vi "MicroZed Test Bench.vi"() -> ()   [LabVIEW 2014]
uses:
  Controls/NamedError.ctl
  Controls/PC Data.ctl
  Controls/MicroZed Config Op Mode.ctl
  Controls/MicroZed Config.ctl
panel:
  out "Version String":string
  in  "PC Config":T1={"AC Voltage SP"=0.0, "AC Current SP"=0.0, "Frequency SP"=60.0, "DC Voltage SP"=0.0, "Op Mode SP"=enum."Shutdown (Reset)", "Clear Faults SP"=0} {"Clear Faults SP" format="%01x"; "DC Voltage SP" min=300 max=550 format="%2.1f"; "Frequency SP" min=45 max=65 format="%2.1f"; "AC Current SP" min=-500 max=500 format="%2.1f"; "AC Voltage SP" min=0 max=132 format="%2.1f"}
  out "PC Data":T3 {"Alarms 2" format="%016b"; "Faults 2" format="%016b"; "Alarms 1" format="%016b"; "Faults 1" format="%016b"; "Contactor FB" format="%.0b"; "DC Voltage SP" format="%2.1f"; "Clear Faults SP" format="%.0b"; "Neutral Current" format="%2.1f"; "AC Current - L2" format="%2.1f"; "AC Voltage - L2" format="%2.1f"; "Temperature" format="%2.1f"; "DC Voltage" format="%2.1f"; "AC Current SP" format="%2.1f"; "AC Voltage SP" format="%2.1f"; "Frequency SP" format="%2.1f"; "AC Frequency" format="%2.1f"; "AC Current - L1" format="%2.1f"; "AC Voltage- L1" format="%2.1f"}
  out "Counter":i32
  in  "port (502)":u16=1502
  in  "address":string="192.168.1.231"
  in  "Clear Error":bool
  out "Slave Error":T4
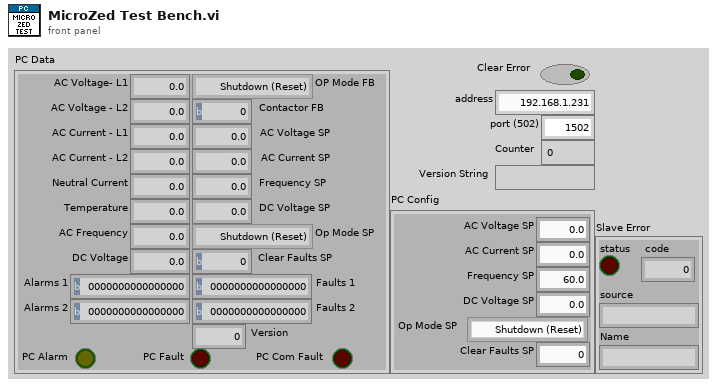
[diagram p1: front panel]
types:
  T1 = typedef "MicroZed Config.ctl" = cluster{"AC Voltage SP":sgl, "AC Current SP":sgl, "Frequency SP":sgl, "DC Voltage SP":sgl, "Op Mode SP":T2, "Clear Faults SP":i16}
  T2 = typedef "MicroZed Config Op Mode.ctl" = enum16{"Shutdown (Reset)", "Startup", "Idle", "Voltage Mode", "Current Mode", "Fault", "OL Voltage (Debug)", "No Data"}
  T3 = typedef "PC Data.ctl" = cluster{"AC Voltage- L1":dbl, "AC Voltage - L2":dbl, "AC Current - L1":dbl, "AC Current - L2":dbl, "Neutral Current":dbl, "Temperature":dbl, "AC Frequency":dbl, "DC Voltage":dbl, "AC Voltage SP":dbl, "AC Current SP":dbl, "Frequency SP":dbl, "Op Mode SP":T2, "Clear Faults SP":u16, "PC Com Fault":bool, "PC Fault":bool, "DC Voltage SP":dbl, "OP Mode FB":T2, "Contactor FB":u16, "Faults 1":u16, "Alarms 1":u16, "Faults 2":u16, "Alarms 2":u16, "PC Alarm":bool, "Version":u16}
  T4 = typedef "NamedError.ctl" = cluster{"status":bool, "code":i32, "source":string, "Name":string}
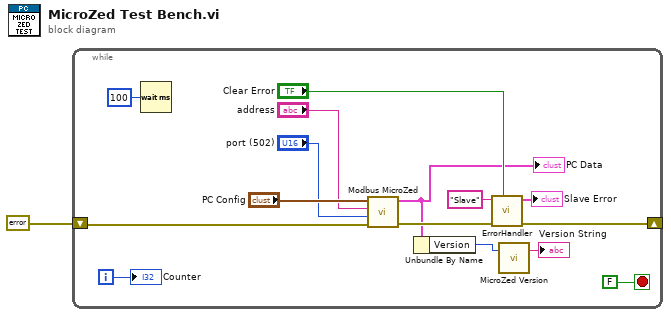
[diagram p0: block diagram]
diagram:
  n1 = while {
    shift-right: [w15] -> _
    shift-left: errorcluster {"status"=FALSE, "code"=0, "source"=""} ("Error Out") -> [w14]
    i -> [w10]
    stop <- FALSE stop-if-true
    n2 = Wait (ms)(milliseconds to wait=u32 100) -> ()  [unwired: 1 out]
    n3 = call "Modbus MicroZed.vi"("Error In"=w14, "port (502)"="port (502)", "address"="address", "PC Config"="PC Config") -> ("Error Out"=w16:errorcluster, "PC Data"=w4:T3)  [unwired: 6 in]
    "PC Data" <- w4
    n4 = Unbundle By Name(w4) -> ("Version"=w3:u16)
    n5 = call "ErrorHandler.vi"("Clear Error"="Clear Error", "Error In"=w16, "Name"="Slave") -> ("Error Out"=w15:errorcluster, "Named Error Out"=→"Slave Error":T4)  [unwired: 5 in]
    n6 = call "MicroZed Version.vi"("Version Numeric"=w3) -> ("Version String"=→"Version String":string)  [unwired: 2 in]
    "Counter" <- w10
  }
